vi "PID test.vi"() -> ()   [LabVIEW 2017]
uses:
  <vilib>/Platform/TimedLoop/XDataNode/timing_clust.ctl
  <vilib>/Platform/TimedLoop/XDataNode/nitl_modes.ctl
  <vilib>/Platform/TimedLoop/XDataNode/wakeup.ctl
  <vilib>/myRIO/Common/Instrument Driver Framework/myRIO v1.0/Encoder/typedefs/Encoder Signal Mode.ctl
  <vilib>/myRIO/Instrument Drivers/Onboard IO/Encoder/typedefs/Encoder Reference.ctl
  <vilib>/myRIO/Common/Instrument Driver Framework/Utilities/typedefs/myRIO Generic Hardware Reference.ctl
  <vilib>/myRIO/Common/Instrument Driver Framework/Utilities/typedefs/Hardware Version Enum.ctl
  <vilib>/myRIO/Common/Instrument Driver Framework/Utilities/typedefs/myRIO v1.0 Reference.ctl
  <vilib>/myRIO/Common/Instrument Driver Framework/Utilities/typedefs/Generic FPGA Reference.ctl
  <vilib>/myRIO/Common/Instrument Driver Framework/myRIO v1.0/Encoder/typedefs/Encoder Channels Enum.ctl
  <vilib>/myRIO/Common/Instrument Driver Framework/myRIO v1.0/Encoder/typedefs/Encoder Configuration v1.0.ctl
  <vilib>/userdefined/High Color/nirio_resource_hc.ctl
  <vilib>/myRIO/Common/Instrument Driver Framework/Utilities/vis/Is FPGA Ref Available.vi
  <vilib>/myRIO/Common/Instrument Driver Framework/myRIO v1.0/Encoder/vis/myRIO v1.1 Open Encoder.vi
  <vilib>/myRIO/Instrument Drivers/Onboard IO/Encoder/vis/Read.vi
  <vilib>/myRIO/Common/Instrument Driver Framework/Utilities/vis/Validate Channels.vi
  <vilib>/myRIO/Common/Instrument Driver Framework/myRIO v1.0/Encoder/vis/myRIO v1.0 Reserve Encoder.vi
  <vilib>/myRIO/Common/Instrument Driver Framework/myRIO v1.0/UART/vis/myRIO v1.0 Close UART.vi
  <vilib>/myRIO/Common/Instrument Driver Framework/myRIO v1.0/Encoder/vis/myRIO v1.0 Build MUX Configuration Encoder.vi
  <vilib>/myRIO/Common/Instrument Driver Framework/myRIO v1.0/Resource Manager/vis/myRIO v1.0 Reserve Channel List.vi
  <vilib>/myRIO/Common/Instrument Driver Framework/myRIO v1.0/Resource Manager/vis/myRIO v1.0 Create Configuration List.vi
  <vilib>/myRIO/Common/Instrument Driver Framework/myRIO v1.0/Resource Manager/vis/myRIO v1.0 Reserve Channel.vi
  <vilib>/myRIO/Common/Instrument Driver Framework/myRIO v1.0/Resource Manager/vis/myRIO v1.0 Unreserve Channel.vi
  <vilib>/myRIO/Common/Instrument Driver Framework/myRIO v1.0/Resource Manager/vis/myRIO v1.0 Build Mutex Name.vi
  Inputs.vi
  <vilib>/Utility/VariantDataType/GetNumericInfo.vi
  <vilib>/Utility/error.llb/Error Cluster From Error Code.vi
  <vilib>/myRIO/Common/Instrument Driver Framework/myRIO v1.0/myRIO v1.1 Open.vi
  <vilib>/myRIO/Common/Instrument Driver Framework/Utilities/vis/IO Manager.vi
  <vilib>/myRIO/Common/Instrument Driver Framework/Utilities/vis/Configuration Manager.vi
  <vilib>/myRIO/Common/Instrument Driver Framework/myRIO v1.0/Resource Manager/vis/myRIO v1.0 Configure IO.vi
  <vilib>/myRIO/Common/Instrument Driver Framework/myRIO v1.0/myRIO v1.0 Close.vi
  <vilib>/myRIO/Common/Instrument Driver Framework/myRIO v1.0/Encoder/vis/myRIO v1.0 Configure Encoder.vi
  <vilib>/myRIO/Common/Instrument Driver Framework/myRIO v1.0/Encoder/vis/myRIO v1.0 Read Encoder.vi
  <vilib>/myRIO/Common/Instrument Driver Framework/Utilities/vis/FPGA Ref Manager.vi
  <vilib>/myRIO/Common/Instrument Driver Framework/myRIO v1.0/myRIO v1.0 Reset FPGA.vi
  <vilib>/myRIO/Common/Instrument Driver Framework/myRIO v1.0/IRQ/vis/myRIO v1.0 IRQ Info FGV.vi
  <vilib>/myRIO/Common/Instrument Driver Framework/myRIO v1.0/IRQ/vis/myRIO v1.0 Timer IRQ Info FGV.vi
  <vilib>/myRIO/Common/Instrument Driver Framework/myRIO v1.0/IRQ/vis/myRIO v1.0 ISR Agent.vi
  <vilib>/platform/TimedLoop/XDataNode/XDataNode.xnode
  <vilib>/myRIO/Express VI/Onboard IO/Encoder/Encoder Express VI.xnode
  <vilib>/myRIO/Instrument Drivers/Onboard IO/Encoder/vis/myRIO Encoder Open.xnode
  <vilib>/myRIO/Common/Instrument Driver Framework/myRIO v1.0/Encoder/typedefs/Encoder Count Direction Enum.ctl
  <vilib>/myRIO/Instrument Drivers/Onboard IO/Encoder/Encoder.lvlib
  <vilib>/Platform/TimedLoop/XDataNode/XDNodeRunTimeDep.lvlib
  <vilib>/myRIO/Instrument Drivers/Utilities/Utilities.lvlib
panel:
  in  "Vp":dbl
  in  "Vy":dbl
  in  "Vx":dbl
  out "error out":errorcluster
  in  "Stop":bool
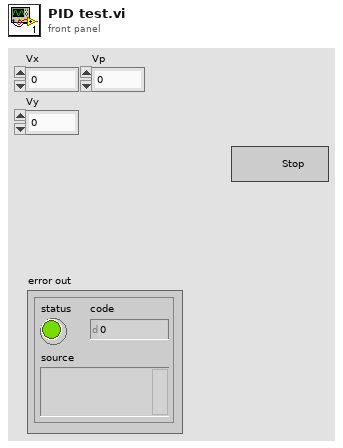
[diagram p1: front panel]
types:
  T1 = typedef "XDNodeRunTimeDep.lvlib/timing_clust.ctl" = cluster{"Expected End [f-1]":u64, "Actual End [f-1]":u64, "Finished Late? [f-1]":bool, "Expected End [i-1]":u64, "Actual End [i-1]":u64, "Finished Late? [i-1]":bool, "Expected Start [i]":u64, "Actual Start [i]":u64, "Expected Start [f]":u64, "Actual Start [f]":u64, "Source Name":string, "Structure Name":string, "Period":i64, "Deadline":i64, "Offset":i64, "Start":i64, "Priority":i32, "Timeout":i32, "Mode":T2, "Wakeup Reason":T3, "Error":errorcluster, "Source Type":string, "Secondary Source Type":string, "Global End Time":u64, "Global Start Time":u64, "Frame Duration":u64, "Iteration Duration":u64, "Assigned CPU":i32, "I/O Scan Engine Mode":u32}
  T2 = typedef "XDNodeRunTimeDep.lvlib/nitl_modes.ctl" = enum32{"No Change", "Process missed periods, maintain original phase", "Discard missed periods, maintain original phase", "Process missed periods, ignore original phase", "Discard missed periods, ignore original phase"}
  T3 = typedef "XDNodeRunTimeDep.lvlib/wakeup.ctl" = enum32{"Normal", "Aborted", "Asynchronous wakeup", "Timing source error", "Timed loop error", "Timeout"}
  T4 = typedef "Encoder.lvlib/Encoder Reference.ctl" = cluster{"myRIO Reference":T5, "Encoder Channels Enum":T9}
  T5 = typedef "myRIO Generic Hardware Reference.ctl" = cluster{"myRIO Model":T6, "myRIO Hardware Reference":T7}
  T6 = typedef "Hardware Version Enum.ctl" = enum16{"Unknown", "myRIO-1900", "myRIO-1950", "roboRIO", "NI ELVIS RIO CM"}
  T7 = typedef "myRIO v1.0 Reference.ctl" = cluster{"Generic FPGA Reference":T8, "Allow multiple opens":bool}
  T8 = typedef "Generic FPGA Reference.ctl" = refnum<k20>
  T9 = typedef "Encoder Channels Enum.ctl" = enum16{"Not Connected", "C/ENC0", "C/ENC1", "A/ENC", "B/ENC", "DIO/ENC0", "DIO/ENC1", "DIO/ENC2", "DIO/ENC3", "DIO/ENC4"}
  T10 = typedef "Encoder Signal Mode.ctl" = enum16{"Quadrature phase signal", "Step and direction signal"}
  T11 = typedef "nirio_resource_hc.ctl" = tag
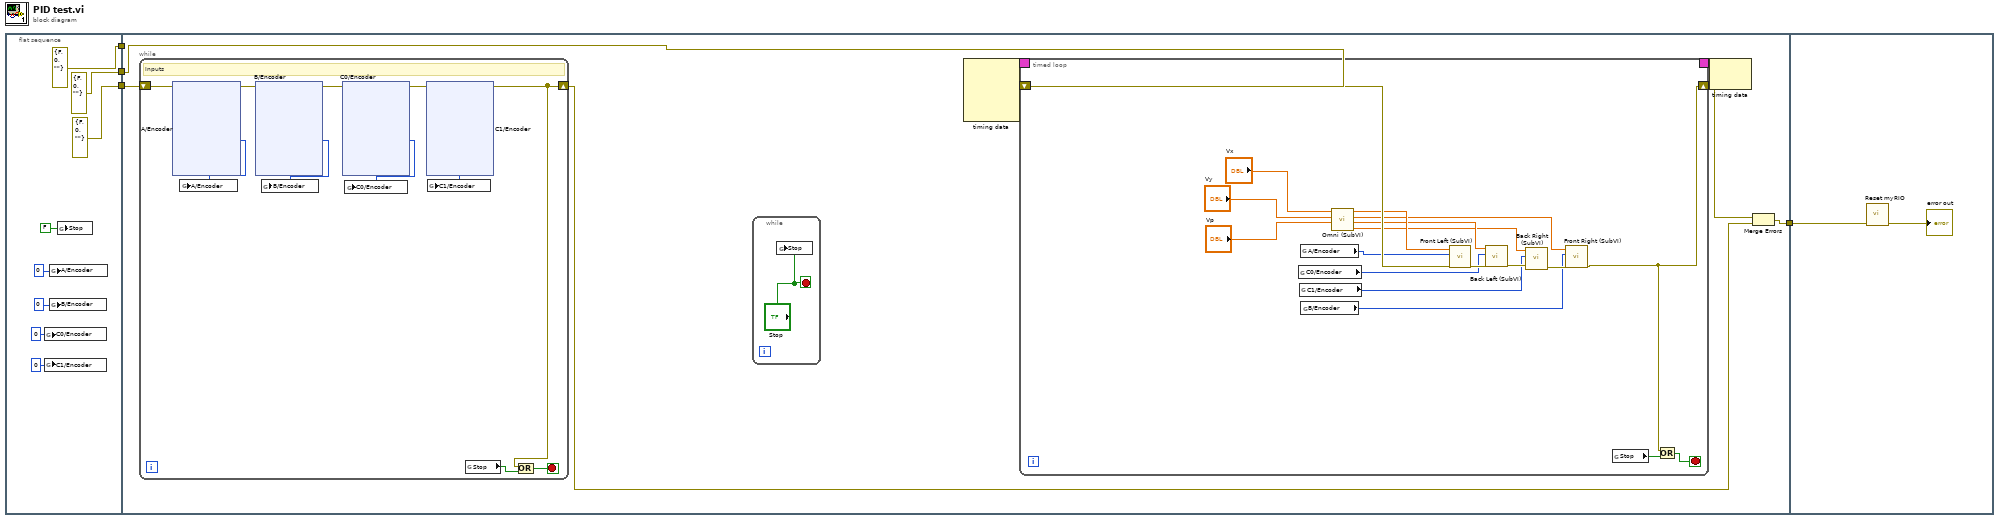
[diagram p0: block diagram]
diagram:
  n1 = flat-sequence {
    tunnel: [errorcluster {"status"=FALSE, "code"=0, "source"=""} ("error in (no error)")] -> w4
    tunnel: [errorcluster {"status"=FALSE, "code"=0, "source"=""} ("error in (no error)")] -> w3
    tunnel: [errorcluster {"status"=FALSE, "code"=0, "source"=""} ("error in (no error)")] -> w2
    tunnel: w4 -> [w19]
    tunnel: [w15] -> w1
    tunnel: w3 -> [_]
    tunnel: w2 -> [w14]
    tunnel: w1 -> [w238]
    frame #0 {
      # "Initialize"
      n2 = global write "Inputs.vi" "C0/Encoder"(0 ("A/Encoder")) -> ()
      n3 = global write "Inputs.vi" "C1/Encoder"(0 ("A/Encoder")) -> ()
      n4 = global write "Inputs.vi" "A/Encoder"(0 ("A/Encoder")) -> ()
      n5 = global write "Inputs.vi" "B/Encoder"(0 ("A/Encoder")) -> ()
      n6 = global write "Inputs.vi" "Stop"(FALSE ("Stop")) -> ()
    }
    frame #1 {
      n7 = while {
        shift-right: [w43] -> w13
        shift-left: w19 -> [w50]
        stop <- w44 stop-if-true
        # "Inputs"
        n8 = xnode "A/Encoder"("error in (no error)"=w50) -> ("Counter Value"=w53:i32, "error out"=w51:errorcluster)  [unwired: 1 in, 2 out]
        n9 = global write "Inputs.vi" "A/Encoder"(w53) -> ()
        n10 = xnode "B/Encoder"("error in (no error)"=w51) -> ("Counter Value"=w52:i32, "error out"=w47:errorcluster)  [unwired: 1 in, 2 out]
        n11 = global write "Inputs.vi" "B/Encoder"(w52) -> ()
        n12 = xnode "C0/Encoder"("error in (no error)"=w47) -> ("Counter Value"=w49:i32, "error out"=w46:errorcluster)  [unwired: 1 in, 2 out]
        n13 = global write "Inputs.vi" "C0/Encoder"(w49) -> ()
        n14 = xnode "C1/Encoder"("error in (no error)"=w46) -> ("Counter Value"=w48:i32, "error out"=w43:errorcluster)  [unwired: 1 in, 2 out]
        n15 = global write "Inputs.vi" "C1/Encoder"(w48) -> ()
        n16 = global read "Inputs.vi" "Stop"() -> (w45:bool)
        n17 = Or(x=w43, y=w45) -> (x .or. y?=w44:bool)
      }
      n18 = while {
        stop <- "Stop" stop-if-true
        n19 = global write "Inputs.vi" "Stop"("Stop") -> ()
      }
      n20 = node-c288() -> (w18:T1)  [unwired: 4 in]
      n21 = timed-loop {
        timing: w18 -> [_]
        timing-out: [_] -> w17
        shift-right: [w29] -> w16
        shift-left: w14 -> [w35]
        stop <- w36 stop-if-true
        n22 = global read "Inputs.vi" "C0/Encoder"() -> (w32:i32)
        n23 = global read "Inputs.vi" "C1/Encoder"() -> (w28:i32)
        n24 = global read "Inputs.vi" "A/Encoder"() -> (w34:i32)
        n25 = global read "Inputs.vi" "B/Encoder"() -> (w27:i32)
        n26 = call "Omni (SubVI).vi"("Vp"="Vp", "Vy"="Vy", "Vx"="Vx") -> ("Back_Right"=w23:dbl, "Back_Left"=w24:dbl, "Front_Right"=w25:dbl, "Front_Left"=w26:dbl)  [unwired: 4 in]
        n27 = call "Front Left (SubVI).vi"("setpoint"=w26, "Counter Value"=w34, "error in"=w35) -> ("error out"=w33:errorcluster)  [unwired: 6 in, 1 out]
        n28 = call "Back Left (SubVI).vi"("error in"=w33, "Counter Value"=w32, "setpoint"=w24) -> ("error out"=w31:errorcluster)  [unwired: 7 in, 1 out]
        n29 = call "Back Right (SubVI).vi"("error in"=w31, "Counter Value"=w28, "setpoint"=w23) -> ("error out"=w30:errorcluster)  [unwired: 7 in, 1 out]
        n30 = call "Front Right (SubVI).vi"("error in"=w30, "Counter Value"=w27, "setpoint"=w25) -> ("error out"=w29:errorcluster)  [unwired: 7 in, 1 out]
        n31 = global read "Inputs.vi" "Stop"() -> (w37:bool)
        n32 = Or(x=w29, y=w37) -> (x .or. y?=w36:bool)
      }
      n33 = node-c288(w17) -> ()  [unwired: 1 out]
      n34 = Merge Errors(w16, w13) -> (w15:errorcluster)
    }
    frame #2 {
      # "Close"
      n35 = call <vilib>:"Reset myRIO.vi"("error in (no error)"=w238) -> ("error out"=→"error out":errorcluster)  [unwired: 10 in]
    }
  }
